vi "CThread False CRef Constants.vi"() -> (2 "Boolean CRef Address":u16)   [LabVIEW 2012, in "CThread.lvlib"]
uses:
  CThread.lvlib
  CRef/CRef.lvlib
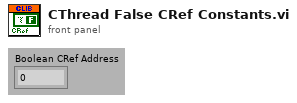
[diagram p1: front panel]
types:
  T1 = typedef "CRef.lvlib/Boolean CReference.ctl" = cluster{"Boolean CRef Address":u16, "Type":enum8{"Null", "Boolean", "U8", "I8", "U16", "I16", "U32", "I32", "U64", "I64", "Single", "Double", "Extended", "CSG", "CDB", "CXT", "Boolean(Def)"}}
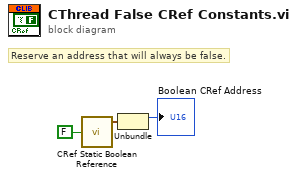
[diagram p0: block diagram]
diagram:
  # "Reserve an address that will always be false."
  n1 = call "CRef Static Boolean Reference.vi"("Initial Value (False)"=FALSE) -> ("Boolean CReference"=w2:T1)  [unwired: 4 in]
  n2 = Unbundle(w2) -> ("Boolean CRef Address"=→"Boolean CRef Address":u16)  [unwired: 1 out]
